vi "CC Calculate Focus offset from filter wheels.vi"(8 "error in (no error)":errorcluster, 11 "Filter positions":i32[](array[numeric])) -> (0 "error out":errorcluster, 3 "New focus offset":dbl)   [LabVIEW 2024]
uses:
  Logging/CC enum Current Values Action.ctl
  hk-channel-class/hk-channel-class/HK Table/HK Table.lvclass
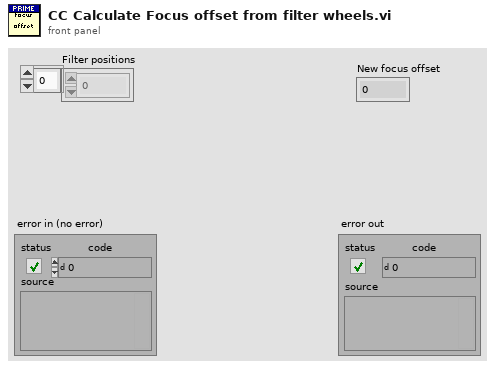
[diagram p1: front panel]
types:
  T1 = typedef "CC enum Current Values Action.ctl" = enum16{"Init", "Write Item", "Write Array", "Read Item", "Read Array", "Read All", "Add Channels", "New File", "Add Message", "Get Current Values", "Close"}
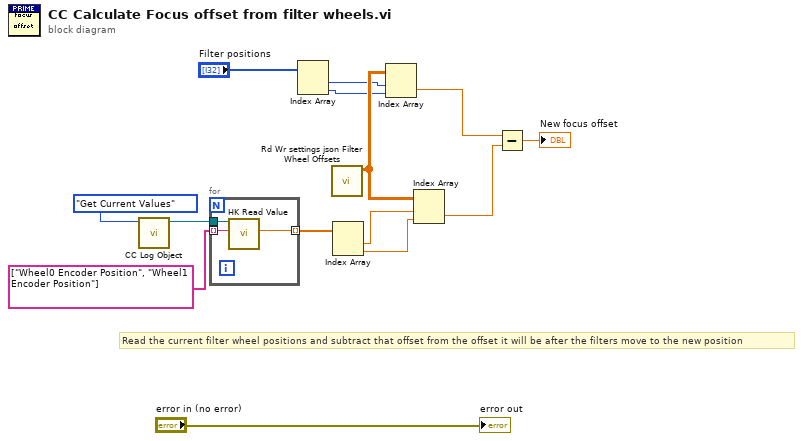
[diagram p0: block diagram]
diagram:
  # "Read the current filter wheel positions and subtract that offset from the offset it will be after the filters move to the new position"
  n1 = call "CC Log Object.vi"("Action"=CC_enum_Current_Values_Action."Get Current Values") -> ("HK Channel out"=w12:refnum<class "HK Table.lvclass">)  [unwired: 8 in, 2 out]
  n2 = for {
    tunnel: w12 -> [w17]
    tunnel: string[] ["Wheel0 Encoder Position", "Wheel1 Encoder Position"] -> [w16] mode=indexing
    tunnel: [w15] -> w10 mode=indexing
    n3 = call-dynamic "HK Read Value.vi"("Channel Name"=w16, "HK Channel in"=w17) -> ("Value"=w15:dbl)  [unwired: 4 in, 5 out]
  }
  n4 = Index Array(array="Filter positions") -> (element #1=w6:i32, element #2=w5:i32)  [unwired: 2 in]
  n5 = call "Rd Wr settings json Filter Wheel Offsets.vi"() -> ("Offsets"=w7:dbl[][])  [unwired: 10 in, 1 out]
  n6 = Index Array(array=w10) -> (element #1=w4:dbl, element #2=w3:dbl)  [unwired: 2 in]
  n7 = Index Array(array=w7, index (row)=w6, index (col)=w5) -> (element=w2:dbl)
  n8 = Index Array(array=w7, index (row)=w4, index (col)=w3) -> (element=w1:dbl)
  n9 = Subtract(x=w2, y=w1) -> (x-y=→"New focus offset":dbl)
  "error out" <- "error in (no error)"
